vi "Hardware Test.vi"() -> ()   [LabVIEW 2020]
uses:
  <vilib>/Platform/TimedLoop/XDataNode/timing_clust.ctl
  <vilib>/Platform/TimedLoop/XDataNode/nitl_modes.ctl
  <vilib>/Platform/TimedLoop/XDataNode/wakeup.ctl
  <vilib>/MakerHub/LINX/Private/Device/Type Defs/Pulse Polarity.ctl
  <vilib>/MakerHub/LINX/Public/Peripherals/Digital/Digital Write N Chans.vi
  <vilib>/MakerHub/LINX/Public/Peripherals/Digital/Digital Read N Chans.vi
  <vilib>/MakerHub/LINX/Public/Peripherals/PWM/PWM Set Duty Cycle 1 Chan.vi
  <vilib>/MakerHub/LINX/Private/Local IO/LinxDigitalWrite.vi
  <vilib>/MakerHub/LINX/Public/Utilities/Check Channel.vi
  <vilib>/MakerHub/LINX/Private/Local IO/LinxDigitalRead.vi
  <vilib>/MakerHub/LINX/Public/Utilities/Open Serial.vi
  <vilib>/MakerHub/LINX/Public/Sensors/Motion/Servo/Servo Open N Channels.vi
  <vilib>/MakerHub/LINX/Private/Utilties/Generate Error.vi
  <vilib>/MakerHub/LINX/Public/Peripherals/PWM/PWM Set Duty Cycle N Chans.vi
  <vilib>/MakerHub/LINX/Public/Sensors/Motion/Servo/Servo Set Pulse Width One Channel.vi
  <vilib>/MakerHub/LINX/Public/Sensors/Motion/Servo/Servo Close N Channels.vi
  <vilib>/platform/TimedLoop/XDataNode/XDataNode.xnode
  <vilib>/MakerHub/LINX/LMH-LINX.lvlib
  <vilib>/MakerHub/LINX/Public/Sensors/Motion/Servo/Servo.lvlib
  <vilib>/Platform/TimedLoop/XDataNode/XDNodeRunTimeDep.lvlib
  <vilib>/MakerHub/LINX/Private/Device/Device.lvlib
panel:
  out "Blue Color":bool
  out "Green Color":bool
  out "Red Color":bool
  out "Blue Freq":u32
  out "Green Freq":u32
  out "Red Freq":u32
  in  "LED Values":bool[](array[boolean])=[FALSE, FALSE, FALSE, FALSE]
  out "Sensor Value":bool[](array[boolean])
  in  "Digital Sensors":u8[](array[numeric])=[30, 32, 34, 36, 38, 50, 52]
  in  "Duty Cycle":dbl(knob)=31.0 scale=0.0..100.0
  in  "PWM Channel":u8=2
  in  "LED Indicators & \nMotor Enable":u8[](array[numeric])=[49, 51, 53, 24]
  in  "Servo Angle  1":u16(slide)=115 scale=0.0..180.0
  in  "Servo Angle  2":u16(slide)=84 scale=0.0..180.0
  in  "Servo Angle  3":u16(slide)=82 scale=0.0..180.0
  in  "stop":bool
  in  "Servo Slider 2":u8=4
  in  "Servo Slider 1":u8=5
  out "Device Name":string
  in  "Serial Port":refnum<visa-resource-name>="N/A"
  in  "Servo Magazine":u8=3
  # "PROGRAM FOR HARDWARE TEST"
  # "Trainer MPS Sorting Based Arduino"
  # "SENSOR & LED"
  # "COLOR DETECT"
  # "SERVO"
  # "MOTOR"
  # "Index Array Digital Sensors\n\n0. IR Stack Magazine\n1. IR Black/White Check\n2. IR Slider 1\n3. IR Slider 2\n4. IR Slider 3\n5. Inductive Proximity \n6. Push Button"
  # "Mechatronics Engineering 2nd Generation - Vocational High School 2 Bojonegoro"
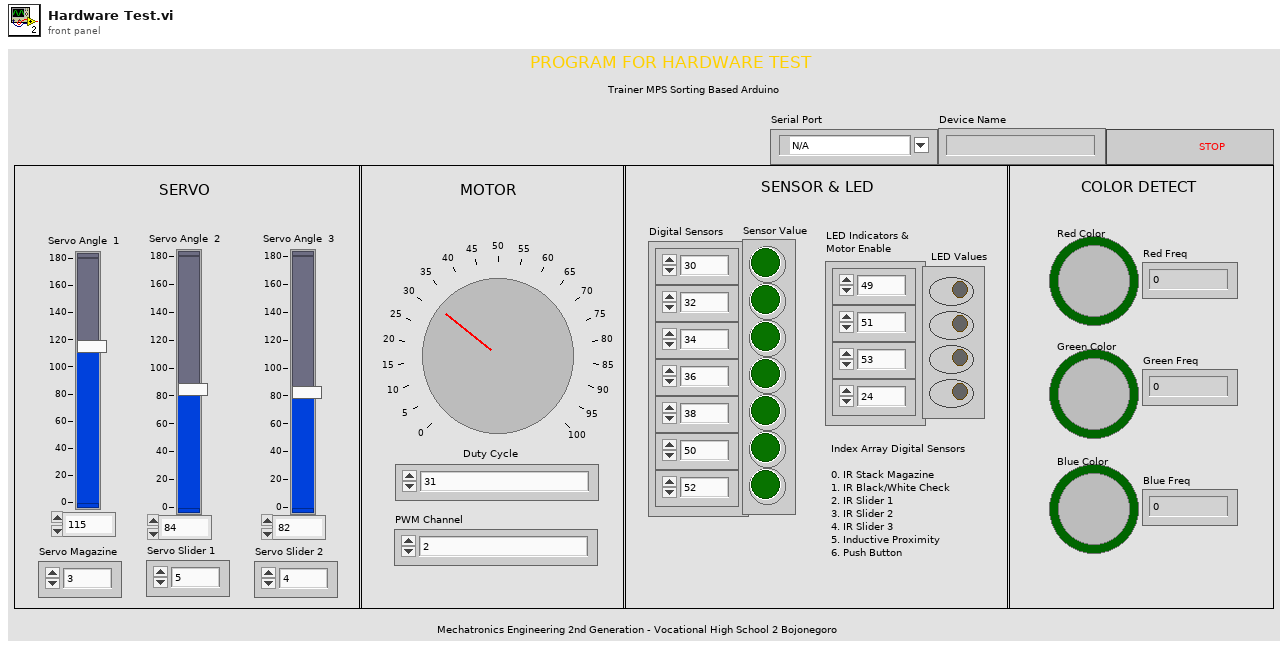
[diagram p1: front panel]
types:
  T1 = typedef "LMH-LINX.lvlib/LINX Ref.ctl" = cluster{"IO":T2, "Interface":T3, "LINX Device Config":T4}
  T2 = typedef "LMH-LINX.lvlib/Platform.ctl" = enum16{"Remote", "Local"}
  T3 = typedef "LMH-LINX.lvlib/Interface.ctl" = enum16{"Serial", "TCP"}
  T4 = typedef "LMH-LINX.lvlib/Device.lvlib/LINX Device Config.ctl" = cluster{"Interface":T3, "COM Port":refnum<visa-resource-name>, "TCP Configuration":T5, "Device Family":u8, "Device ID":u8, "Device Name":string, "TCP Ref":refnum<k5>, "Channels":T6}
  T5 = typedef "LMH-LINX.lvlib/Device.lvlib/TCP Config.ctl" = cluster{"IP Address":string, "Port":u16}
  T6 = typedef "LMH-LINX.lvlib/Channels.ctl" = cluster{"DI":u8[], "DO":u8[], "AI":u8[], "AO":u8[], "PWM":u8[], "QE":u8[], "UART":u8[], "I2C 2":u8[], "SPI":u8[], "CAN":u8[], "Servo":u8[], "AI Ref (V)":dbl, "AI Resolution (Bits)":u8, "AO Ref (V)":dbl, "AO Resolution (Bits)":u8}
  T7 = typedef "XDNodeRunTimeDep.lvlib/timing_clust.ctl" = cluster{"Expected End [f-1]":u64, "Actual End [f-1]":u64, "Finished Late? [f-1]":bool, "Expected End [i-1]":u64, "Actual End [i-1]":u64, "Finished Late? [i-1]":bool, "Expected Start [i]":u64, "Actual Start [i]":u64, "Expected Start [f]":u64, "Actual Start [f]":u64, "Source Name":string, "Structure Name":string, "Period":i64, "Deadline":i64, "Offset":i64, "Start":i64, "Priority":i32, "Timeout":i32, "Mode":T8, "Wakeup Reason":T9, "Error":errorcluster, "Source Type":string, "Secondary Source Type":string, "Global End Time":u64, "Global Start Time":u64, "Frame Duration":u64, "Iteration Duration":u64, "Assigned CPU":i32, "I/O Scan Engine Mode":u32}
  T8 = typedef "XDNodeRunTimeDep.lvlib/nitl_modes.ctl" = enum32{"No Change", "Process missed periods, maintain original phase", "Discard missed periods, maintain original phase", "Process missed periods, ignore original phase", "Discard missed periods, ignore original phase"}
  T9 = typedef "XDNodeRunTimeDep.lvlib/wakeup.ctl" = enum32{"Normal", "Aborted", "Asynchronous wakeup", "Timing source error", "Timed loop error", "Timeout"}
  T10 = typedef "LMH-LINX.lvlib/Device.lvlib/Pulse Polarity.ctl" = enum8{"Active Low", "Active High"}
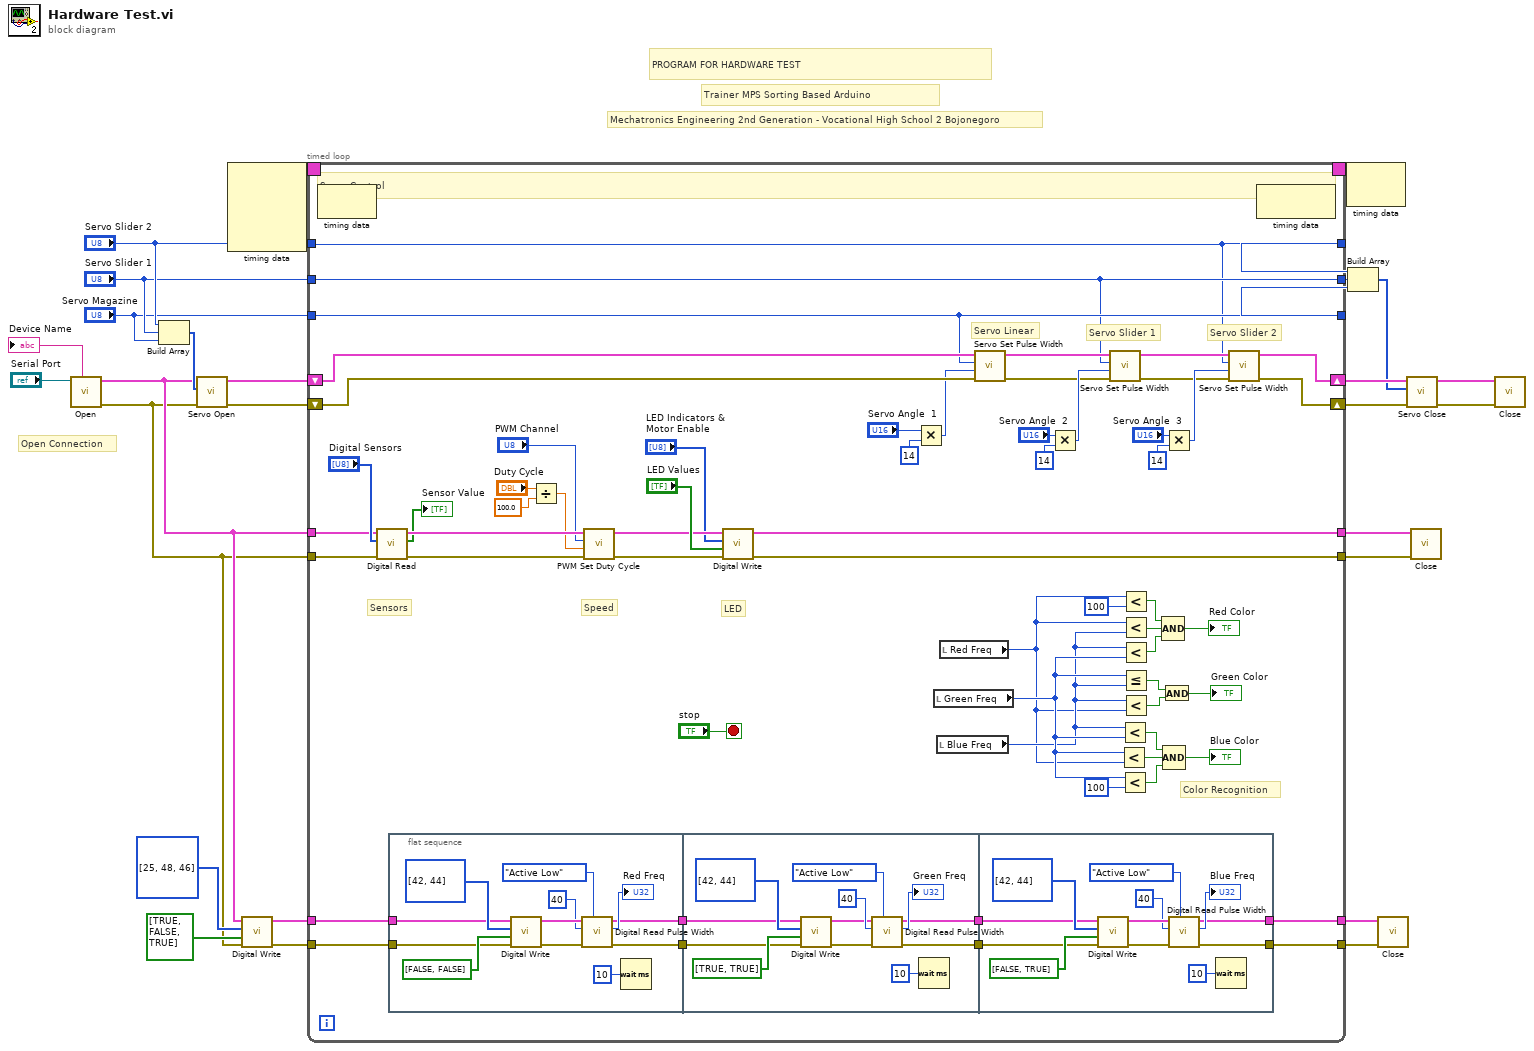
[diagram p0: block diagram]
diagram:
  # "Mechatronics Engineering 2nd Generation - Vocational High School 2 Bojonegoro"
  # "Open Connection"
  # "Trainer MPS Sorting Based Arduino"
  # "PROGRAM FOR HARDWARE TEST"
  n1 = call-poly <vilib>:"Open.vi"("Serial Port"="Serial Port") -> ("Error Out"=w1:errorcluster, "Device Name"=→"Device Name":string, "LINX Resource"=w2:T1)  [unwired: 8 in]
  n2 = Build Array("Servo Slider 2", "Servo Slider 1", "Servo Magazine") -> (w22:u8[])
  n3 = call-poly <vilib>:"Servo Open.vi"("Error In"=w1, "Servo Channels"=w22, "LINX Resource"=w2) -> ("Error Out"=w3:errorcluster, "LINX Resource"=w4:T1)  [unwired: 7 in]
  n4 = node-c288() -> (w28:T7)  [unwired: 4 in]
  n5 = call-poly <vilib>:"Digital Write.vi"("Error In"=w1, "Values"=bool[] [TRUE, FALSE, TRUE], "DO Channels"=u8[] [25, 48, 46], "LINX Resource"=w2) -> ("Error Out"=w6:errorcluster, "LINX Resource"=w5:T1)  [unwired: 6 in]
  n6 = timed-loop {
    tunnel: "Servo Magazine" -> [w74]
    shift-right: [w76] -> w26
    shift-left: w4 -> [w89]
    shift-right: [w75] -> w25
    shift-left: w3 -> [w87]
    tunnel: "Servo Slider 1" -> [w73]
    tunnel: "Servo Slider 2" -> [w72]
    tunnel: [w72] -> w18
    tunnel: [w73] -> w17
    tunnel: [w74] -> w16
    timing: w28 -> [_]
    timing-out: [_] -> w27
    tunnel: w2 -> [w56]
    tunnel: w1 -> [w55]
    tunnel: [w29] -> w12
    tunnel: [w54] -> w11
    tunnel: [w49] -> w10
    tunnel: [w48] -> w9
    tunnel: w6 -> [w47]
    tunnel: w5 -> [w46]
    stop <- "stop" stop-if-true
    # "Color Recognition"
    # "Servo Linear"
    # "LED"
    # "Speed"
    # "Sensors"
    # "Servo Slider 2"
    # "Servo Slider 1"
    # "Servo Control"
    n7 = node-c288() -> ()  [unwired: 1 in, 1 out]
    n8 = call-poly <vilib>:"Digital Read.vi"("Error In"=w55, "DI Channels"="Digital Sensors", "LINX Resource"=w56) -> ("Error Out"=w68:errorcluster, "Values"=→"Sensor Value":bool[], "LINX Resource"=w67:T1)  [unwired: 6 in]
    n9 = flat-sequence {
      tunnel: w46 -> [w97]
      tunnel: w47 -> [w96]
      tunnel: [w92] -> w53
      tunnel: [w91] -> w52
      tunnel: w53 -> [w106]
      tunnel: w52 -> [w105]
      tunnel: [w103] -> w51
      tunnel: [w102] -> w50
      tunnel: w51 -> [w117]
      tunnel: w50 -> [w116]
      tunnel: [w115] -> w49
      tunnel: [w114] -> w48
      frame #0 {
        n10 = call-poly <vilib>:"Digital Write.vi"("Error In"=w96, "Values"=bool[] [FALSE, FALSE], "DO Channels"=u8[] [42, 44], "LINX Resource"=w97) -> ("Error Out"=w95:errorcluster, "LINX Resource"=w98:T1)  [unwired: 6 in]
        n11 = call <vilib>:"Digital Read Pulse Width.vi"("Incoming Pulse Polarity (Active High)"=Pulse_Polarity."Active Low", "Error In"=w95, "DI Channel"=u8 40, "LINX Resource"=w98) -> ("Error Out"=w91:errorcluster, "Pulse Width (uS)"=→"Red Freq":u32, "LINX Resource"=w92:T1)  [unwired: 5 in]
        n12 = Wait (ms)(milliseconds to wait=u32 10) -> ()  [unwired: 1 out]
      }
      frame #1 {
        n13 = call-poly <vilib>:"Digital Write.vi"("Error In"=w105, "Values"=bool[] [TRUE, TRUE], "DO Channels"=u8[] [42, 44], "LINX Resource"=w106) -> ("Error Out"=w111:errorcluster, "LINX Resource"=w110:T1)  [unwired: 6 in]
        n14 = call <vilib>:"Digital Read Pulse Width.vi"("Incoming Pulse Polarity (Active High)"=Pulse_Polarity."Active Low", "Error In"=w111, "DI Channel"=u8 40, "LINX Resource"=w110) -> ("Error Out"=w103:errorcluster, "Pulse Width (uS)"=→"Green Freq":u32, "LINX Resource"=w102:T1)  [unwired: 5 in]
        n15 = Wait (ms)(milliseconds to wait=u32 10) -> ()  [unwired: 1 out]
      }
      frame #2 {
        n16 = call-poly <vilib>:"Digital Write.vi"("Error In"=w117, "Values"=bool[] [FALSE, TRUE], "DO Channels"=u8[] [42, 44], "LINX Resource"=w116) -> ("Error Out"=w120:errorcluster, "LINX Resource"=w121:T1)  [unwired: 6 in]
        n17 = call <vilib>:"Digital Read Pulse Width.vi"("Incoming Pulse Polarity (Active High)"=Pulse_Polarity."Active Low", "Error In"=w120, "DI Channel"=u8 40, "LINX Resource"=w121) -> ("Error Out"=w114:errorcluster, "Pulse Width (uS)"=→"Blue Freq":u32, "LINX Resource"=w115:T1)  [unwired: 5 in]
        n18 = Wait (ms)(milliseconds to wait=u32 10) -> ()  [unwired: 1 out]
      }
    }
    n19 = Divide(x="Duty Cycle", y=100.0) -> (x/y=w63:dbl)
    n20 = call-poly <vilib>:"PWM Set Duty Cycle.vi"("Error In"=w68, "Duty Cycle (0-1)"=w63, "PWM Channel"="PWM Channel", "LINX Resource"=w67) -> ("Error Out"=w58:errorcluster, "LINX Resource"=w59:T1)  [unwired: 6 in]
    n21 = call-poly <vilib>:"Digital Write.vi"("Error In"=w58, "Values"="LED Values", "DO Channels"="LED Indicators & \nMotor Enable", "LINX Resource"=w59) -> ("Error Out"=w54:errorcluster, "LINX Resource"=w29:T1)  [unwired: 6 in]
    n22 = Multiply(x="Servo Angle  1", y=u16 14) -> (x*y=w70:u16)
    n23 = local read "Green Freq"() -> (w36:u32)
    n24 = local read "Blue Freq"() -> (w35:u32)
    n25 = local read "Red Freq"() -> (w30:u32)
    n26 = call-poly <vilib>:"Servo Set Pulse Width.vi"("Error In"=w87, "Pulse Width (uS)"=w70, "Servo Channel"=w74, "LINX Resource"=w89) -> ("Error Out"=w77:errorcluster, "LINX Resource"=w79:T1)  [unwired: 6 in]
    n27 = Multiply(x="Servo Angle  2", y=u16 14) -> (x*y=w84:u16)
    n28 = call-poly <vilib>:"Servo Set Pulse Width.vi"("Error In"=w77, "Pulse Width (uS)"=w84, "Servo Channel"=w73, "LINX Resource"=w79) -> ("Error Out"=w78:errorcluster, "LINX Resource"=w80:T1)  [unwired: 6 in]
    n29 = Less?(x=w36, y=w30) -> (x < y?=w38:bool)
    n30 = Less?(x=w35, y=w36) -> (x < y?=w37:bool)
    n31 = Less?(x=w36, y=u32 100) -> (x < y?=w39:bool)
    n32 = Less?(x=w30, y=u32 100) -> (x < y?=w42:bool)
    n33 = Less?(x=w30, y=w35) -> (x < y?=w40:bool)
    n34 = Less?(x=w35, y=w36) -> (x < y?=w41:bool)
    n35 = Less Or Equal?(x=w36, y=w35) -> (x <= y?=w33:bool)
    n36 = Less?(x=w35, y=w30) -> (x < y?=w34:bool)
    n37 = Compound Arithmetic op=AND(w42, w40, w41) -> (→"Red Color":bool)
    n38 = And(x=w33, y=w34) -> (x .and. y?=→"Green Color":bool)
    n39 = Compound Arithmetic op=AND(w37, w38, w39) -> (→"Blue Color":bool)
    n40 = Multiply(x="Servo Angle  3", y=u16 14) -> (x*y=w81:u16)
    n41 = call-poly <vilib>:"Servo Set Pulse Width.vi"("Error In"=w78, "Pulse Width (uS)"=w81, "Servo Channel"=w72, "LINX Resource"=w80) -> ("Error Out"=w75:errorcluster, "LINX Resource"=w76:T1)  [unwired: 6 in]
    n42 = node-c288() -> ()  [unwired: 1 in, 1 out]
  }
  n43 = node-c288(w27) -> ()  [unwired: 1 out]
  n44 = Build Array(w18, w17, w16) -> (w15:u8[])
  n45 = call <vilib>:"Close.vi"("Error In"=w9, "LINX Resource"=w10) -> ()  [unwired: 9 in, 1 out]
  n46 = call-poly <vilib>:"Servo Close.vi"("Error In"=w25, "Servo Channels"=w15, "LINX Resource"=w26) -> ("Error Out"=w13:errorcluster, "LINX Resource"=w14:T1)  [unwired: 7 in]
  n47 = call <vilib>:"Close.vi"("Error In"=w11, "LINX Resource"=w12) -> ()  [unwired: 9 in, 1 out]
  n48 = call <vilib>:"Close.vi"("Error In"=w13, "LINX Resource"=w14) -> ()  [unwired: 9 in, 1 out]
